vi "joystick to robot.vi"(0 "Refnum in":refnum<k1>, 1 "id":u32, 7 "max_v_tang":dbl=1.0 format="%#_13g", 9 "max_v_norm":dbl=1.0 format="%#_13g", 11 "error in (no error)":errorcluster, 12 "max_v_ang":dbl=3.0 format="%#_13g") -> (3 "RobotArray":T1[](array[typedef]), 4 "Refnum out":refnum<k1>, 6 "v_norm":dbl format="%0.2f", 10 "v_tang":dbl format="%0.2f", 14 "v_ang":dbl format="%0.2f", 15 "error out":errorcluster)   [LabVIEW 2020]
uses:
  Communication_class/Paths/Convert AI Robot to Robot Command Folder/grSim/grSim Robot Command.ctl
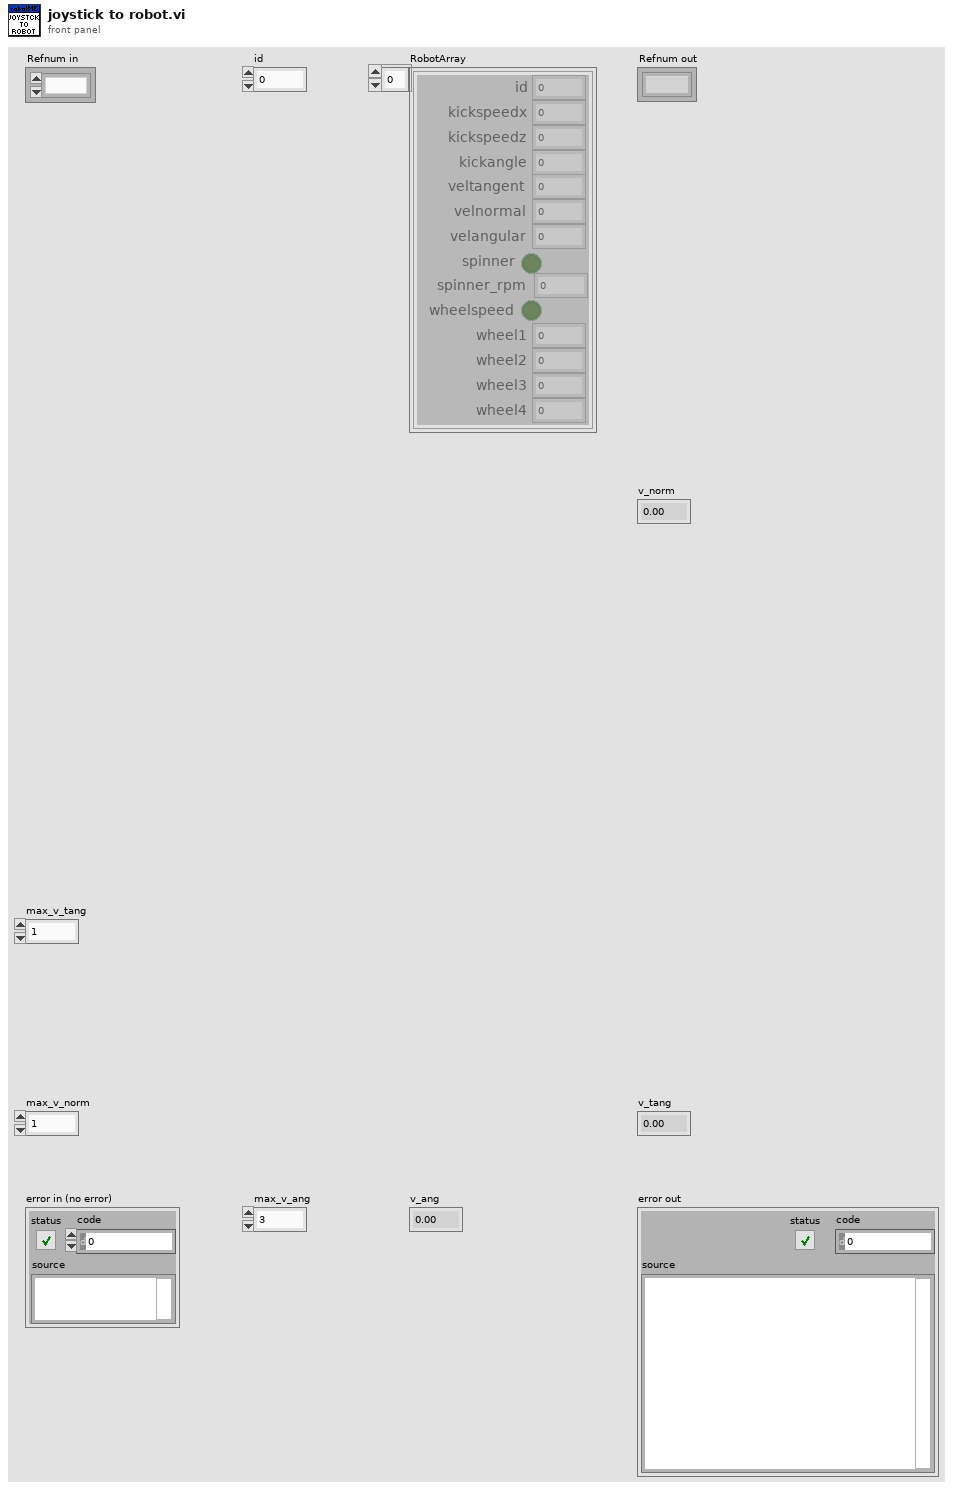
[diagram p1: front panel]
types:
  T1 = typedef "grSim Robot Command.ctl" = cluster{"id":u32, "kickspeedx":sgl, "kickspeedz":sgl, "veltangent":sgl, "velnormal":sgl, "velangular":sgl, "spinner":bool, "wheelspeed":bool, "wheel1":sgl, "wheel2":sgl, "wheel3":sgl, "wheel4":sgl, "kickangle":sgl, "spinner_rpm":sgl}
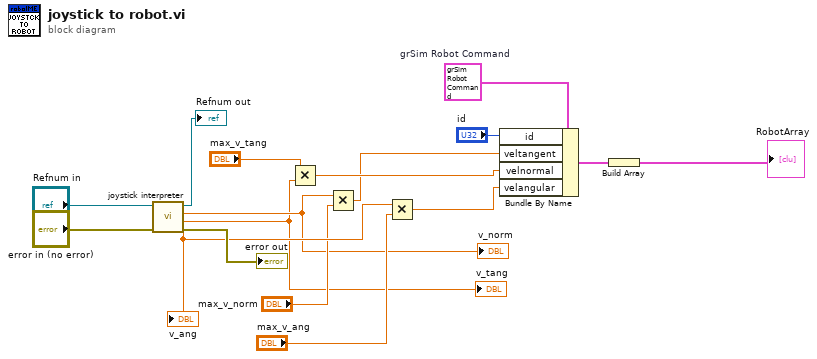
[diagram p0: block diagram]
diagram:
  w1 = T1 {"id"=0, "kickspeedx"=0.0, "kickspeedz"=0.0, "veltangent"=0.0, "velnormal"=0.0, "velangular"=0.0, "spinner"=FALSE, "wheelspeed"=FALSE, "wheel1"=0.0, "wheel2"=0.0, "wheel3"=0.0, "wheel4"=0.0, "kickangle"=0.0, "spinner_rpm"=0.0}  # grSim Robot Command
  n1 = call "joystick interpreter.vi"("error in (no error)"="error in (no error)", "Refnum in"="Refnum in") -> ("error out"=→"error out":errorcluster, "v_tang"=w9:dbl, "v_norm"=w10:dbl, "Refnum out"=→"Refnum out":refnum<k1>, "v_ang"=w13:dbl)  [unwired: 5 in]
  "v_norm" <- w10
  "v_tang" <- w9
  "v_ang" <- w13
  n2 = Multiply(x="max_v_tang", y=w9) -> (x*y=w17:dbl)
  n3 = Multiply(x=w10, y="max_v_norm") -> (x*y=w16:dbl)
  n4 = Multiply(x=w13, y="max_v_ang") -> (x*y=w14:dbl)
  n5 = Bundle By Name(cluster=w1, "id"="id", "veltangent"=w16, "velnormal"=w17, "velangular"=w14) -> (w6:T1)
  n6 = Build Array(w6) -> (→"RobotArray":T1[])
